vi "VI.open_module_lua.vi"(5 "LuaVIEW reference":T1) -> (15 "error out":errorcluster)   [LabVIEW 2012]
doc: "Opens the module at the specified path and initialises it. This should cause the module to set its functions as part of the specified table. If no table is specified (an empty string) or \"_G\" is specified, the functions are set in the global namespace of your script.\n\nLike <a href=\"#VI.open\"><code>VI.open()</code></a>, this function returns a VI object. Since the VI object is prepared for calling, it cannot be run nor executed. After opening the module, it is advisable to immediately add a cleanup that <a href=\"#VI.close\">closes</a> the returned VI object. After closing the module, its functions can no longer be called.\n\nWhen the path is relative, the module will be searched for relative to the directory containing the calling task's main script. If the module is not found there, or if the calling script is not a task, the module will be searched for relative to the resource base path. When running as a built application, the application executable will also be searched. When a VI with the specified name is already in memory, a reference to that VI is opened irrespective of the path.\n\nWhen the module is implemented as a non-reentrant VI, there is only one dataspace and there can only be one caller at a time. Depending on the implementation of such a module, it may or may not be possible to open and use it from multiple script contexts simultaneously. When the module is a reentrant VI, a new dataspace is created on opening the module. This allows multiple instances of one module to be opened, each with a separate configuration and state. Still, there can only be one caller per instance at any one time. Use a VI template when the full VI state must be instantiated, e.g. for debugging or when the front panel must be visible. When you must call multiple instances of the same module from within the same script, use a different table name for each instance so as to keep their functions separate.\n\nModules are handy for implementing a set of functions that operate on a shared state or a shared resource. They can also be used as a quick and dirty means of implementing related functions without the full bother of creating and documenting multiple LuaVIEW VIs and adding background infrastructure to tie these functions together.\n\nWhen the module contains export functions, any scripts started after opening the module can call those functions. The export functions are registered under the specified export table or as globals when an empty string is specified. When there can be multiple instances of the module, be sure to use a unique name for the export table. Consider choosing a valid Lua variable name as the identifier of the task that opens and manages a module instance and reuse that as the name of the export table. A task's identifier can be retrieved via <a href=\"#task.identifier\"><code>task.identifier()</code></a>\n\nTo configure a module, provide a configuration table. The format of the table varies from module to module and typically reflects a LabVIEW cluster. When the module does not require configuration, the table must be omitted. When the module provides a default configuration, the entire table or named elements in the table can be omitted and will be substituted for by the default data.\nParameters:\nstr:path, path to the module VI or template.\nstr:table, table to be filled with the module functions. The global table is used when an empty string is specified.\nstr:exptab, table to register export functions under. Must be unique per instance.\n[tab:config], optional configuration table to pass to the module. \nResults:\nobj:vi, VI object of the module.\nErrors:\nSpecified module not found.\nConfiguration table is missing (when required by module).\nConfiguration table has an invalid format.\nUnable to open module VI reference.\nUnable to initialise module VI, e.g. because its implementation is broken.\nAny errors returned during initialisation."
uses:
  typedefs/t_LuaVIEW Reference.ctl
  typedefs/et_LuaVIEW CIN Actions.ctl
  subvis/private/LuaVIEW Pull (path).vi
  subvis/private/LuaVIEW Push (refnum).vi
  subvis/private/LuaVIEW Push (object).vi
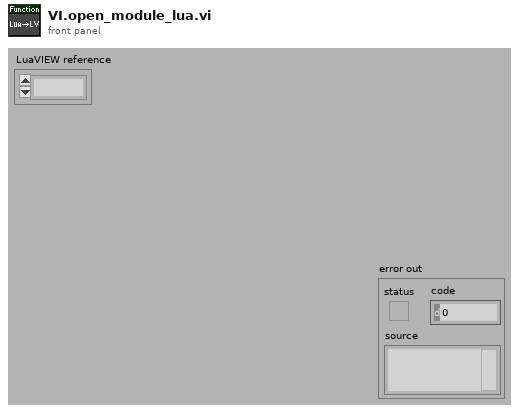
[diagram p1: front panel]
types:
  T1 = typedef "t_LuaVIEW Reference.ctl" = refnum<k1>
  T2 = typedef "et_LuaVIEW CIN Actions.ctl" = enum16{"checksynopsis", "_open", "_registerpublic", "_registerexport", "__never_an_error_result_ns", "luaversion", "cinversion", "_totals", "_taskcount", "pathological", "_unregnextpublic", "registryusecount", "__per_state_actions", "regsetprivate", "regsetindex", "regsetmodule", "_revokeexports", "_usepublic", "prepare", "compile", "execute", "call", "unregstaterefs", "_close", "pullboolean", "pullnumber", "pullI8", "pullU8", "pullI16", "pullU16", "pullI32", "pullU32", "pullobject", "pullrefnum", "pullstring", "pullflat", "pushflat", "pushobject", "getattribute", "setattribute", "stacktostring", "_startyieldtest", "_endyieldtest", "_pollprintbuffer", "__never_an_error_result_ps", "_pollexport", "setclone", "forcecleanup", "gettop", "clearstack", "insert", "pushboolean", "pushnumber", "pushrefnum", "pushstring", "pushnil", "pushvalue", "gettaskref", "settaskref"}
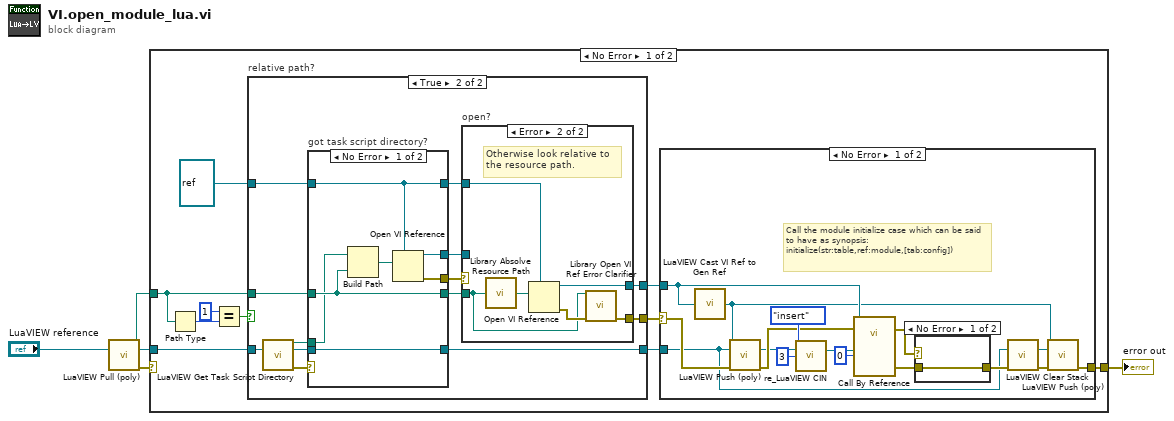
[diagram p0: block diagram]
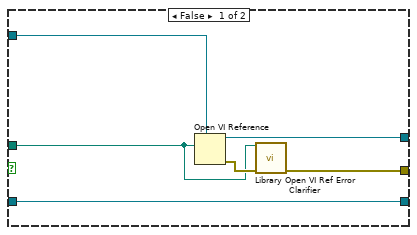
[diagram p4: hidden frame]
diagram:
  n1 = call-poly "LuaVIEW Pull (poly).vi"("LuaVIEW reference in"="LuaVIEW reference") -> ("path"=w4:path, "LuaVIEW reference out"=w2:T1, "error out"=w1:errorcluster)  [unwired: 12 in]
  n2 = case shown="No Error" w1 {
    selector: w1 -> [_ w73]
    tunnel: [w9 w73] -> w5
    tunnel: w4 -> [w7 _]
    tunnel: w2 -> [w12 _]
    frame No Error {
      n3 = Path Type(1:w7) -> (0:w15:i16)
      n4 = Equal?(x=i16 1, y=w15) -> (x = y?=w13:bool)
      n5 = case "relative path?" shown="True" w13 {
        tunnel: w12 -> [w40 w44]
        tunnel: [w40 w51] -> w11
        tunnel: w7 -> [w38 w53]
        tunnel: [w37 w46] -> w8
        tunnel: [w36 w45] -> w10
        tunnel: refnum<vi> refnum ("module pane") -> [w35 w52]
        frame False {
          n6 = Open VI Reference(type specifier VI Refnum (for type only)=w35, vi path=w38) -> (vi reference=w36:refnum<vi>, error out=w39:errorcluster)  [unwired: 4 in]
          n7 = call "Library Open VI Ref Error Clarifier.vi"("VI path"=w38, "called VI error (no error)"=w39) -> ("error out"=w37:errorcluster)  [unwired: 13 in]
        }
        frame True {
          n8 = call "LuaVIEW Get Task Script Directory.vi"("LuaVIEW reference in"=w44) -> ("task script directory"=w42:path, "LuaVIEW reference out"=w43:T1, "error out"=w41:errorcluster)  [unwired: 12 in]
          n9 = case "got task script directory?" shown="No Error" w41 {
            selector: w41 -> [_ w69]
            tunnel: w53 -> [w66 w71]
            tunnel: w52 -> [w63 w70]
            tunnel: w43 -> [w67 w72]
            tunnel: [w67 w72] -> w51
            tunnel: [w66 w71] -> w48
            tunnel: [w65 w69] -> w50
            tunnel: [w64 _] -> w49
            tunnel: [w63 w70] -> w47
            tunnel: w42 -> [w62 _]
            frame No Error {
              n10 = Build Path(base path=w62, name or relative path=w66) -> (appended path=w68:path)
              n11 = Open VI Reference(type specifier VI Refnum (for type only)=w63, vi path=w68) -> (vi reference=w64:refnum<vi>, error out=w65:errorcluster)  [unwired: 4 in]
            }
            frame Error {
            }
          }
          n12 = case "open?" shown="Error" w50 {
            selector: w50 -> [w54 _]
            tunnel: w49 -> [w55 _]
            tunnel: w48 -> [_ w57]
            tunnel: w47 -> [_ w61]
            tunnel: [w54 w58] -> w46
            tunnel: [w55 w56] -> w45
            frame No Error {
            }
            frame Error {
              # "Otherwise look relative to\nthe resource path."
              n13 = call "Library Absolve Resource Path.vi"("path in"=w57) -> ("absolved path"=w60:path)  [unwired: 14 in]
              n14 = Open VI Reference(type specifier VI Refnum (for type only)=w61, vi path=w60) -> (vi reference=w56:refnum<vi>, error out=w59:errorcluster)  [unwired: 4 in]
              n15 = call "Library Open VI Ref Error Clarifier.vi"("VI path"=w57, "called VI error (no error)"=w59) -> ("error out"=w58:errorcluster)  [unwired: 13 in]
            }
          }
        }
      }
      n16 = case shown="No Error" w8 {
        selector: w8 -> [w28 w34]
        tunnel: w11 -> [w22 _]
        tunnel: w10 -> [w27 _]
        tunnel: [w25 w34] -> w9
        frame No Error {
          # "Call the module initialize case which can be said to have as synopsis:\ninitialize(str:table,ref:module,[tab:config])"
          n17 = call "LuaVIEW Cast VI Ref to Gen Ref.vi"("refnum in"=w27) -> ("refnum out"=w26:refnum<vi>)  [unwired: 14 in]
          n18 = call-poly "LuaVIEW Push (poly).vi"("refnum"=w26, "LuaVIEW reference in"=w22, "error in (no error)"=w28) -> ("LuaVIEW reference out"=w17:T1, "error out"=w18:errorcluster)  [unwired: 11 in]
          n19 = call "re_LuaVIEW CIN.vi"("action"=et_LuaVIEW_CIN_Actions."insert", "LuaVIEW reference in"=w17, "index in"=3) -> ("LuaVIEW reference out"=w16:T1)  [unwired: 6 in, 6 out]
          n20 = call-by-ref "?"(reference=w27, error in=w18, "LuaVIEW reference"=w16, "function index"=0) -> (error out=w31:errorcluster, 15:"error out"=w30:errorcluster)  [unwired: 13 in, 1 out]
          n21 = case shown="No Error" w31 {
            selector: w31 -> [_ w33]
            tunnel: [w32 w33] -> w24
            tunnel: w30 -> [w32 _]
            frame No Error {
            }
            frame Error {
            }
          }
          n22 = call "LuaVIEW Clear Stack.vi"("LuaVIEW reference in"=w22, "error in (no error)"=w24) -> ("LuaVIEW reference out"=w21:T1, "error out"=w23:errorcluster)  [unwired: 12 in]
          n23 = call-poly "LuaVIEW Push (poly).vi"("object refnum"=w26, "LuaVIEW reference in"=w21, "error in (no error)"=w23) -> ("error out"=w25:errorcluster)  [unwired: 11 in, 1 out]
        }
        frame Error {
        }
      }
    }
    frame Error {
    }
  }
  "error out" <- w5
